vi "Get Device Info.vi"(8 "error in (no error)":errorcluster, 11 "Handle":u64) -> (0 "error out":errorcluster, 2 "Device Information":T1 {"Type" items=["FT232B-FT245B", "FT8U232AM-FT8U245AM", "FT8U100AX", "UNKNOWN", "FT2232", "FT232R-FT245R", "FT2232H", "FT4232H", "FT232H"]}, 3 "Handle out":u64)   [LabVIEW 2019, in "D2XX-lv.lvlib"]
doc: "Get device information for an open device."
uses:
  D2XX-lv.lvlib
  <instrlib>/_D2XX/D2XX/D2XX.lvlib
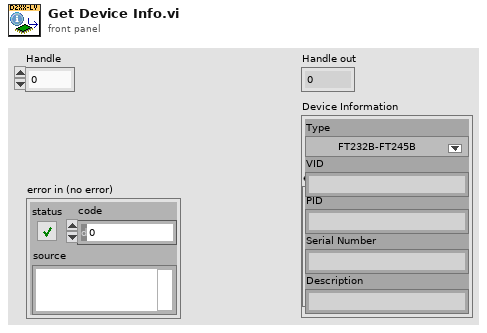
[diagram p1: front panel]
types:
  T1 = cluster{"Type":u32, "VID":string, "PID":string, "Serial Number":string, "Description":string}
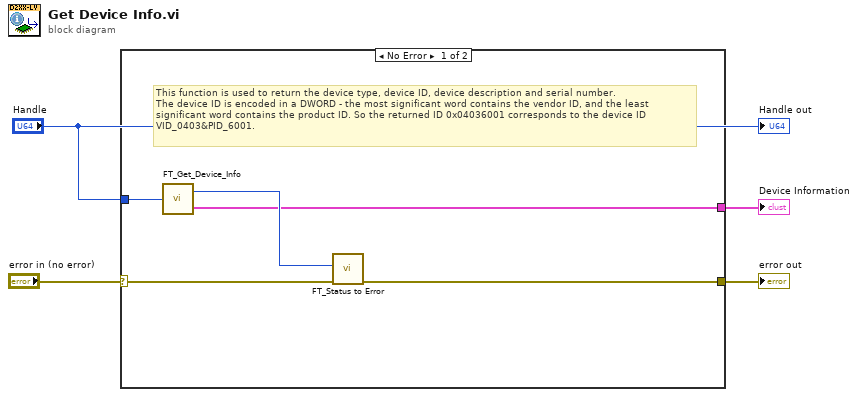
[diagram p0: block diagram]
diagram:
  n1 = case shown="No Error" "error in (no error)" {
    selector: "error in (no error)" -> [w9 w10]
    tunnel: [w5 w10] -> w3
    tunnel: "Handle" -> [w8 _]
    tunnel: [w6 _] -> w1
    frame No Error {
      # "This function is used to return the device type, device ID, device description and serial number.\nThe device ID is encoded in a DWORD - the most significant word contains the vendor ID, and the least\nsignificant word contains the product ID. So the returned ID 0x04036001 corresponds to the device ID\nVID_0403&PID_6001."
      n2 = call <instrlib>:"FT_Get_Device_Info.vi"("Handle"=w8) -> ("FT_Status"=w7:u32, "Device Information"=w6:T1)
      n3 = call "FT_Status to Error.vi"("error in (no error)"=w9, "FT_Status"=w7) -> ("error out"=w5:errorcluster)  [unwired: 9 in]
    }
    frame Error {
    }
  }
  "error out" <- w3
  "Device Information" <- w1
  "Handle out" <- "Handle"
